vi "CRYUnflatten User Equation Cluster.vi"(11 "Flatten user equation cluster string":string) -> (0 "Header info":T2={"Data type"="Data            ", "Version"=1, "Dimensions"=0}, 3 "User Equation Cluster":T1 {"Results axis" items=["x", "y", "z"]; "Input axis" items=["x", "y", "z"]; "Custom unit results array"."dB ref" format="%.2f"; "Custom unit input array"."dB ref" format="%.2f"}, 4 "Error?":bool)   [LabVIEW 2013]
uses:
  Typedef Control/CRYUser Equation Cluster.ctl
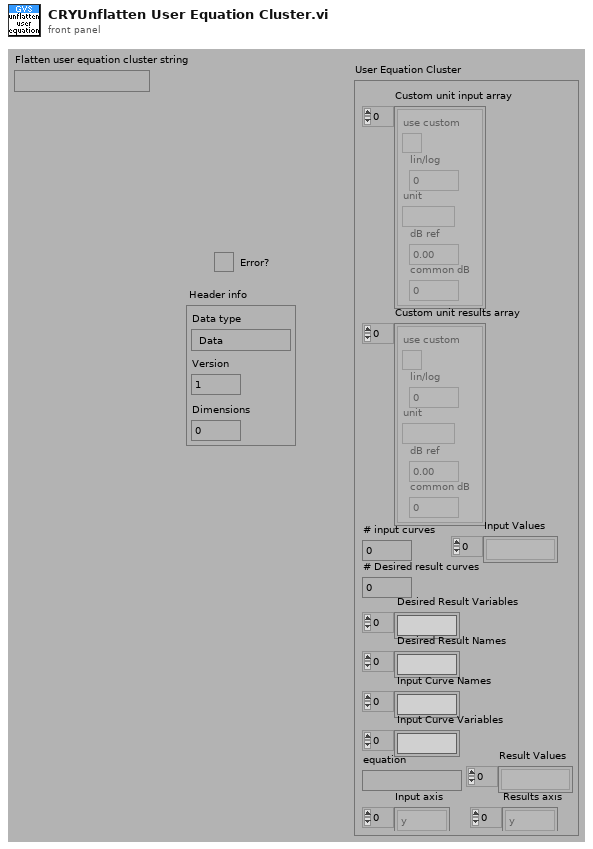
[diagram p1: front panel]
types:
  T1 = typedef "CRYUser Equation Cluster.ctl" = cluster{"Custom unit input array":cluster{"use custom":bool, "lin/log":u16, "unit":string, "dB ref":dbl, "common dB":u16}[], "Custom unit results array ":cluster{"use custom":bool, "lin/log":u16, "unit":string, "dB ref":dbl, "common dB":u16}[], "Desired Result Variables":string[], "Desired Result Names":string[], "Input Curve Names":string[], "Input Curve Variables":string[], "equation":string, "Input axis":u16[], "Results axis":u16[], "# input curves":i32, "# Desired result curves ":i32, "Input Values":string[], "Result Values":string[]}
  T2 = cluster{"Data type":string, "Version":u16, "Dimensions":u8}
  T3 = cluster{"unsigned byte array[0]":u8, "unsigned byte array[1]":u8, "unsigned byte array[2]":u8}
  T4 = cluster{"substring":string, u16, "unsigned byte array[2]":u8}
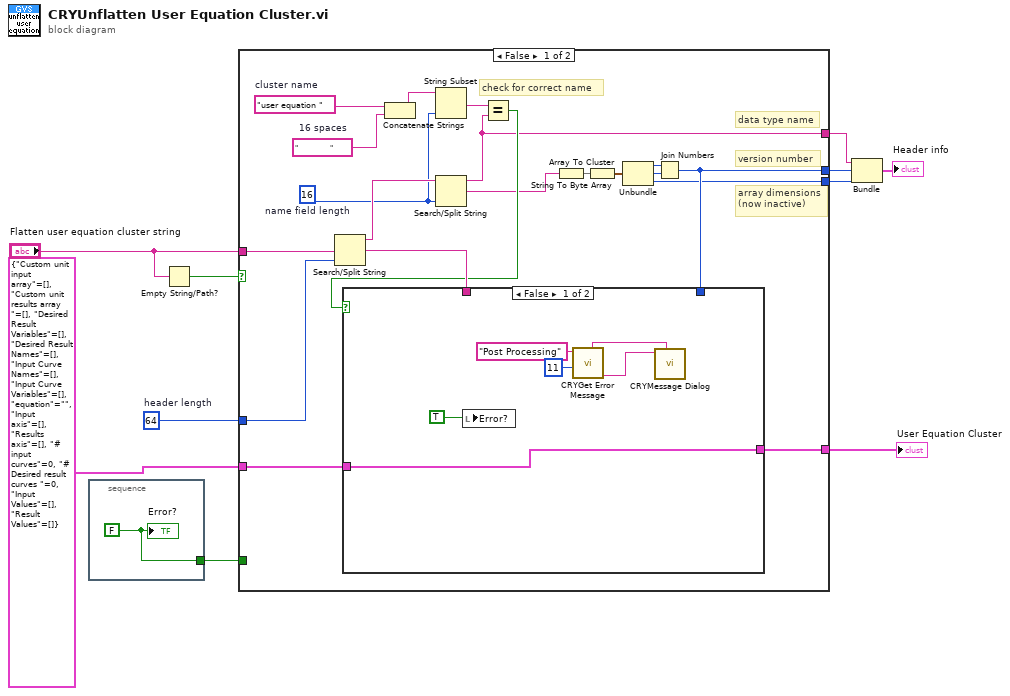
[diagram p0: block diagram]
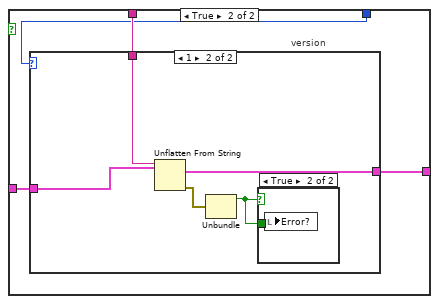
[diagram p2: hidden frame]
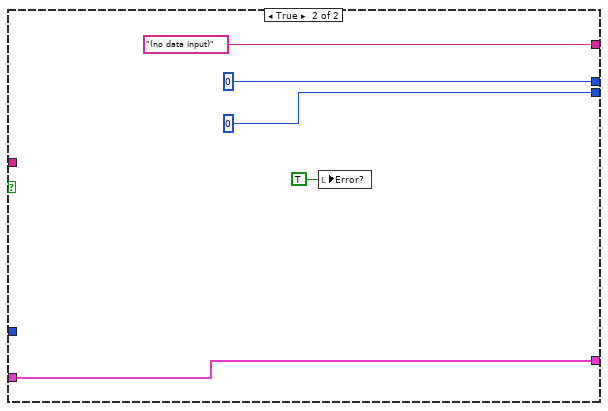
[diagram p5: hidden frame]
diagram:
  w8 = 64  # header length
  n1 = stacked-sequence {
    tunnel: [w11] -> w3
    frame #0 {
      w11 = FALSE
      "Error?" <- w11
    }
  }
  n2 = Empty String/Path?(string/path="Flatten user equation cluster string") -> (empty?=w9:bool)
  n3 = case shown="False" w9 {
    tunnel: "Flatten user equation cluster string" -> [w31 _]
    tunnel: w8 -> [w25 _]
    tunnel: [w22 u16 0] -> w6
    tunnel: [w14 u8 0] -> w7
    tunnel: [w15 "(no data input)" ("substring")] -> w5
    tunnel: w3 -> [_ _]
    tunnel: [w13 w49] -> w1
    tunnel: T1 {"Custom unit input array"=[], "Custom unit results array "=[], "Desired Result Variables"=[], "Desired Result Names"=[], "Input Curve Names"=[], "Input Curve Variables"=[], "equation"="", "Input axis"=[], "Results axis"=[], "# input curves"=0, "# Desired result curves "=0, "Input Values"=[], "Result Values"=[]} ("User Equation Cluster") -> [w12 w49]
    frame False {
      w19 = "                "  # 16 spaces
      w20 = "user equation "  # cluster name
      w17 = 16  # name field length
      # "check for correct name"
      # "array dimensions\n(now inactive)"
      # "version number"
      # "data type name"
      n4 = Search/Split String(string=w31, offset (0)=w25) -> (substring before match=w24:string, match + rest of string=w26:string)  [unwired: 2 out]
      n5 = Concatenate Strings(w20, w19) -> (w18:string)
      n6 = String Subset(string=w18, length (rest)=w17) -> (substring=w16:string)  [unwired: 1 out]
      n7 = Search/Split String(string=w24, offset (0)=w17) -> (substring before match=w15:string, match + rest of string=w21:string)  [unwired: 2 out]
      n8 = Equal?(x=w16, y=w15) -> (x = y?=w23:bool)
      n9 = String To Byte Array(string=w21) -> (unsigned byte array=w30:u8[])
      n10 = Array To Cluster(array=w30) -> (cluster=w29:T3)
      n11 = Unbundle(w29) -> ("unsigned byte array[0]"=w28:u8, "unsigned byte array[1]"=w27:u8, "unsigned byte array[2]"=w14:u8)
      n12 = Join Numbers(hi=w28, lo=w27) -> ((hi.lo)=w22:u16)
      n13 = case shown="False" w23 {
        tunnel: w26 -> [_ w41]
        tunnel: w22 -> [_ w40]
        tunnel: [w36 w39] -> w13
        tunnel: w12 -> [w36 w38]
        frame False {
          n14 = local write "Error?"(TRUE) -> ()
          n15 = call "CRYGet Error Message.vi"("Error No"=11 ("No"), "Kind"="Post Processing") -> ("Message Sub 3"=w32:string, "Window Title"=w33:string)  [unwired: 4 in, 4 out]
          n16 = call "CRYMessage Dialog.vi"("Window Title"=w33, "Message Content"=w32) -> ()  [unwired: 8 in, 2 out]
        }
        frame True {
          n17 = case "version" shown="1" w40 {
            tunnel: w41 -> [_ w47]
            tunnel: [w42 w44] -> w39
            tunnel: w38 -> [w42 w45]
            frame Default {
            }
            frame 1 {
              n18 = Unflatten From String(type=w45, binary string=w47) -> (value=w44:T1, error out=w43:errorcluster)  [unwired: 1 in, 3 out]
              n19 = Unbundle(w43) -> ("status"=w46:bool)  [unwired: 2 out]
              n20 = case shown="True" w46 {
                tunnel: w46 -> [_ w48]
                frame False {
                }
                frame True {
                  n21 = local write "Error?"(w48) -> ()
                }
              }
            }
          }
        }
      }
    }
    frame True {
      n22 = local write "Error?"(TRUE ("Error?")) -> ()
    }
  }
  "User Equation Cluster" <- w1
  n23 = Bundle("substring"=w5, w6, "unsigned byte array[2]"=w7) -> (→"Header info":T4)  [unwired: 1 out]
